vi "TempLoop(SubVI).vi"(5 "CS Configuration 2":T10, 6 "Time Target (s)":dbl, 7 "CS Configuration 1":T10, 8 "error in (no error)":errorcluster, 9 "SPI Configuration in":T7, 11 "LINX Resource in":T1) -> (0 "error out":errorcluster, 1 "Temp2":string, 2 "Temp1":string, 3 "LINX Resource out":T1, 4 "Actual Clock Frequency":u32)   [LabVIEW 2017]
uses:
  <vilib>/MakerHub/LINX/Public/Peripherals/SPI/SPI CS Config.ctl
  <vilib>/MakerHub/LINX/Private/Type Defs/Peripherals/SPI/SPI CS Logic Level.ctl
  <vilib>/MakerHub/LINX/Private/Type Defs/Peripherals/SPI/SPI Configuration.ctl
  <vilib>/MakerHub/LINX/Private/Type Defs/Peripherals/SPI/SPI Bit Order.ctl
  <vilib>/MakerHub/LINX/Private/Type Defs/Peripherals/SPI/SPI Mode.ctl
  <vilib>/MakerHub/LINX/Private/Type Defs/LINX Ref.ctl
  <vilib>/MakerHub/LINX/Private/Type Defs/Platform.ctl
  <vilib>/MakerHub/LINX/Private/Type Defs/Interface.ctl
  <vilib>/MakerHub/LINX/Private/Device/Type Defs/LINX Device Config.ctl
  <vilib>/MakerHub/LINX/Private/Device/Type Defs/TCP Config.ctl
  <vilib>/MakerHub/LINX/Private/Device/Type Defs/Channels.ctl
  Global 1.vi
  <vilib>/MakerHub/LINX/LMH-LINX.lvlib
  <vilib>/MakerHub/LINX/Private/Device/Device.lvlib
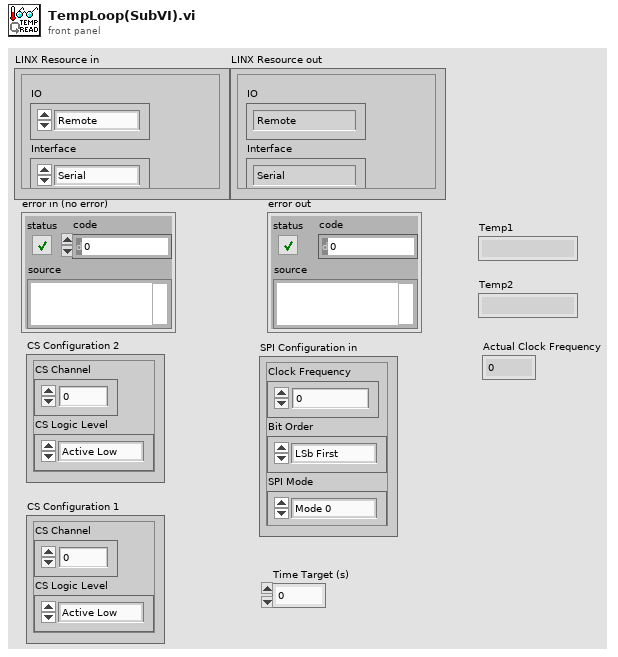
[diagram p1: front panel]
types:
  T1 = typedef "LMH-LINX.lvlib/LINX Ref.ctl" = cluster{"IO":T2, "Interface":T3, "LINX Device Config":T4}
  T2 = typedef "LMH-LINX.lvlib/Platform.ctl" = enum16{"Remote", "Local"}
  T3 = typedef "LMH-LINX.lvlib/Interface.ctl" = enum16{"Serial", "TCP"}
  T4 = typedef "LMH-LINX.lvlib/Device.lvlib/LINX Device Config.ctl" = cluster{"Interface":T3, "COM Port":refnum<visa-resource-name>, "TCP Configuration":T5, "Device Family":u8, "Device ID":u8, "Device Name":string, "TCP Ref":refnum<k5>, "Channels":T6}
  T5 = typedef "LMH-LINX.lvlib/Device.lvlib/TCP Config.ctl" = cluster{"IP Address":string, "Port":u16}
  T6 = typedef "LMH-LINX.lvlib/Channels.ctl" = cluster{"DI":u8[], "DO":u8[], "AI":u8[], "AO":u8[], "PWM":u8[], "QE":u8[], "UART":u8[], "I2C 2":u8[], "SPI":u8[], "CAN":u8[], "Servo":u8[], "AI Ref (V)":dbl, "AI Resolution (Bits)":u8, "AO Ref (V)":dbl, "AO Resolution (Bits)":u8}
  T7 = typedef "LMH-LINX.lvlib/SPI Configuration.ctl" = cluster{"Clock Frequency":u32, "Bit Order":T8, "SPI Mode":T9}
  T8 = typedef "LMH-LINX.lvlib/SPI Bit Order.ctl" = enum8{"LSb First", "MSb First"}
  T9 = typedef "LMH-LINX.lvlib/SPI Mode.ctl" = enum8{"Mode 0", "Mode 1", "Mode 2", "Mode 3"}
  T10 = typedef "LMH-LINX.lvlib/SPI CS Config.ctl" = cluster{"CS Channel":u8, "CS Logic Level":T11}
  T11 = typedef "LMH-LINX.lvlib/SPI CS Logic Level.ctl" = enum8{"Active Low", "Active High"}
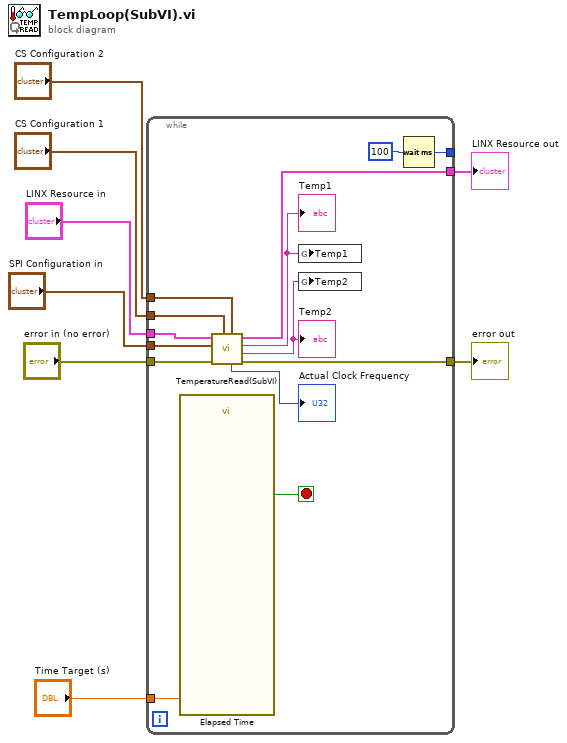
[diagram p0: block diagram]
diagram:
  n1 = while {
    tunnel: "LINX Resource in" -> [w22]
    tunnel: "error in (no error)" -> [w12]
    tunnel: [w21] -> w3
    tunnel: [w20] -> w4
    tunnel: "SPI Configuration in" -> [w19]
    tunnel: "CS Configuration 1" -> [w18]
    tunnel: "CS Configuration 2" -> [w17]
    tunnel: "Time Target (s)" -> [w15]
    tunnel: [w13] -> _
    stop <- w16 stop-if-true
    n2 = call "Elapsed Time"("Time Target (s)"=w15) -> ("Time has Elapsed"=w16:bool)  [unwired: 11 in, 7 out]
    n3 = call "TemperatureRead(SubVI).vi"("CS Configuration 2"=w17, "CS Configuration"=w18, "Error In"=w12, "SPI Configuration"=w19, "LINX Resource"=w22) -> ("Error Out"=w20:errorcluster, "Temp2"=w9:string, "Temp1"=w10:string, "LINX Resource 2"=w21:T1, "Actual Clock Frequency"=→"Actual Clock Frequency":u32)  [unwired: 2 in]
    "Temp1" <- w10
    "Temp2" <- w9
    n4 = global write "Global 1.vi" "Temp1"(w10) -> ()
    n5 = global write "Global 1.vi" "Temp2"(w9) -> ()
    n6 = Wait (ms)(milliseconds to wait=u32 100) -> (millisecond timer value=w13:u32)
  }
  "error out" <- w4
  "LINX Resource out" <- w3
